vi "BufferIndexToPriority.vi"(10 "number of buffers":i32, 11 "buffer index":i32) -> (0 "lowest priority?":bool, 1 "highest priority?":bool, 2 "priority":i32, 3 "buffer index out":i32)   [LabVIEW 2013, in "CLM_PriorityLocalMessage.lvclass"]
uses:
  CLM_PriorityLocalMessage.lvclass
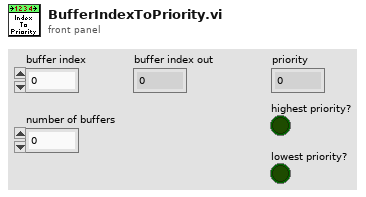
[diagram p1: front panel]
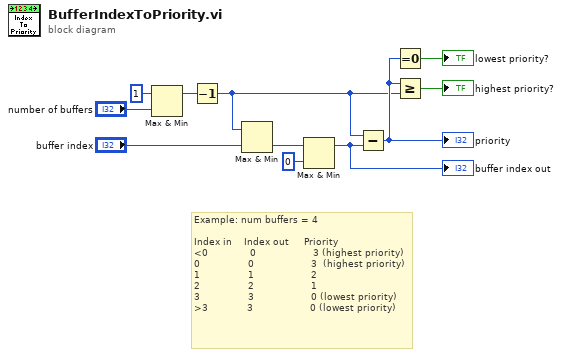
[diagram p0: block diagram]
diagram:
  # "Example: num buffers = 4\n\nIndex in    Index out     Priority\n<0              0                   3 (highest priority)\n0                0                   3  (highest priority)\n1                1                   2\n2                2                   1\n3                3                   0 (lowest priority)\n>3             3                   0 (lowest priority)"
  n1 = Max & Min(x=1, y="number of buffers") -> (max(x,y)=w1:i32)  [unwired: 1 out]
  n2 = Decrement(x=w1) -> (x-1=w6:i32)
  n3 = Max & Min(x=w6, y="buffer index") -> (min(x,y)=w9:i32)  [unwired: 1 out]
  n4 = Max & Min(x=w9, y=0) -> (max(x,y)=w8:i32)  [unwired: 1 out]
  "buffer index out" <- w8
  n5 = Subtract(x=w6, y=w8) -> (x-y=w7:i32)
  "priority" <- w7
  n6 = Equal To 0?(x=w7) -> (x = 0?=→"lowest priority?":bool)
  n7 = Greater Or Equal?(x=w7, y=w6) -> (x >= y?=→"highest priority?":bool)
